vi "ScanrangeX.vi"() -> ()   [LabVIEW 2013]
panel:
  in  "Scanrange X":dbl format="%.2f"
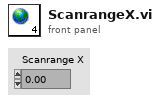
[diagram p1: front panel]
diagram:
